vi "crc8.vi"(4 "Reflect Output? (F)":bool, 6 "Reflect Input? (F)":bool, 8 "Xor Out (0x00)":u8 format="%02x", 9 "Poly (0x07)":u8=7 format="%02x", 10 "Init (0x00)":u8 format="%02x", 11 "Data in":string) -> (3 "CRC-8":u8 format="%02x")   [LabVIEW 2021, in "hashlib.lvlib"]
doc: "Calculates a 8-bit Cyclic Redundancy Check (CRC-8) for various algorithms."
uses:
  hashlib.lvlib
panel:
  # "Data=\"123456789\"\n\nAlgorithm       CRC-8 Poly  Init  RefIn  RefOut XorOut\nCRC-8           0xF4  0x07  0x00  false  false  0x00\nCRC-8/CDMA2000  0xDA  0x9B  0xFF  false  false  0x00\nCRC-8/DARC      0x15  0x39  0x00  true   true   0x00\nCRC-8/DVB-S2    0xBC  0xD5  0x00  false  false  0x00\nCRC-8/EBU       0x97  0x1D  0xFF  true   true   0x00\nCRC-8/I-CODE    0x7E  0x1D  0xFD  false  false  0x00\nCRC-8/ITU       0xA1  0x07  0x00  false  false  0x55\nCRC-8/MAXIM     0xA1  0x31  0x00  true   true   0x00\nCRC-8/ROHC      0xD0  0x07  0xFF  true   true   0x00\nCRC-8/WCDMA     0x25  0x9B  0x00  true   true   0x00\n\nSource: https://crccalc.com/"
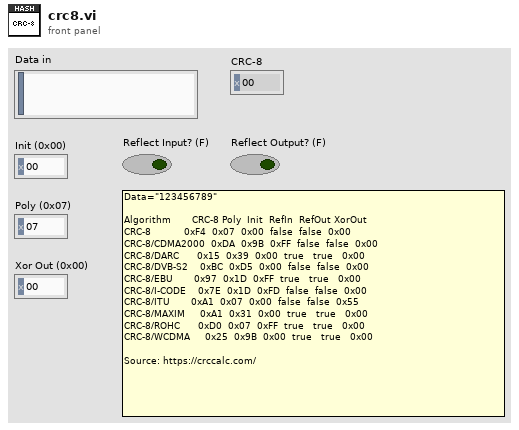
[diagram p1: front panel]
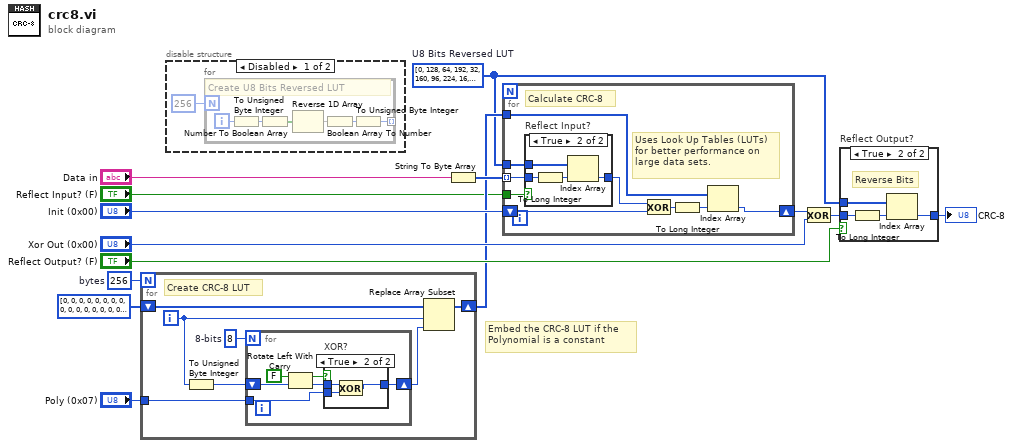
[diagram p0: block diagram]
diagram:
  w1 = u8[] [0, 128, 64, 192, 32, 160, 96, 224, 16, 144, 80, 208, 48, 176, 112, 240, 8, 136, 72, 200, 40, 168, 104, 232, 24, 152, 88, 216, 56, 184, 120, 248, 4, 132, 68, 196, 36, 164, 100, 228, 20, 148, 84, 212, 52, 180, 116, 244, 12, 140, 76, 204, 44, 172, 108, 236, 28, 156, 92, 220, 60, 188, 124, 252, 2, 130, 66, 194, 34, 162, 98, 226, 18, 146, 82, 210, 50, 178, 114, 242, 10, 138, 74, 202, 42, 170, 106, 234, 26, 154, 90, 218, 58, 186, 122, 250, 6, 134, 70, 198, 38, 166, 102, 230, 22, 150, 86, 214, 54, 182, 118, 246, 14, 142, 78, 206, 46, 174, 110, 238, 30, 158, 94, 222, 62, 190, 126, 254, 1, 129, 65, 193, 33, 161, 97, 225, 17, 145, 81, 209, 49, 177, 113, 241, 9, 137, 73, 201, 41, 169, 105, 233, 25, 153, 89, 217, 57, 185, 121, 249, 5, 133, 69, 197, 37, 165, 101, 229, 21, 149, 85, 213, 53, 181, 117, 245, 13, 141, 77, 205, 45, 173, 109, 237, 29, 157, 93, 221, 61, 189, 125, 253, 3, 131, 67, 195, 35, 163, 99, 227, 19, 147, 83, 211, 51, 179, 115, 243, 11, 139, 75, 203, 43, 171, 107, 235, 27, 155, 91, 219, 59, 187, 123, 251, 7, 135, 71, 199, 39, 167, 103, 231, 23, 151, 87, 215, 55, 183, 119, 247, 15, 143, 79, 207, 47, 175, 111, 239, 31, 159, 95, 223, 63, 191, 127, 255]  # U8 Bits Reversed LUT
  w8 = 256  # bytes
  # "Embed the CRC-8 LUT if the\nPolynomial is a constant"
  n1 = for {
    N: w8 -> [_]
    tunnel: "Poly (0x07)" -> [w20]
    shift-right: [w16] -> w3
    shift-left: u8[] [0, 0, 0, 0, 0, 0, 0, 0, 0, 0, 0, 0, 0, 0, 0, 0, 0, 0, 0, 0, 0, 0, 0, 0, 0, 0, 0, 0, 0, 0, 0, 0, 0, 0, 0, 0, 0, 0, 0, 0, 0, 0, 0, 0, 0, 0, 0, 0, 0, 0, 0, 0, 0, 0, 0, 0, 0, 0, 0, 0, 0, 0, 0, 0, 0, 0, 0, 0, 0, 0, 0, 0, 0, 0, 0, 0, 0, 0, 0, 0, 0, 0, 0, 0, 0, 0, 0, 0, 0, 0, 0, 0, 0, 0, 0, 0, 0, 0, 0, 0, 0, 0, 0, 0, 0, 0, 0, 0, 0, 0, 0, 0, 0, 0, 0, 0, 0, 0, 0, 0, 0, 0, 0, 0, 0, 0, 0, 0, 0, 0, 0, 0, 0, 0, 0, 0, 0, 0, 0, 0, 0, 0, 0, 0, 0, 0, 0, 0, 0, 0, 0, 0, 0, 0, 0, 0, 0, 0, 0, 0, 0, 0, 0, 0, 0, 0, 0, 0, 0, 0, 0, 0, 0, 0, 0, 0, 0, 0, 0, 0, 0, 0, 0, 0, 0, 0, 0, 0, 0, 0, 0, 0, 0, 0, 0, 0, 0, 0, 0, 0, 0, 0, 0, 0, 0, 0, 0, 0, 0, 0, 0, 0, 0, 0, 0, 0, 0, 0, 0, 0, 0, 0, 0, 0, 0, 0, 0, 0, 0, 0, 0, 0, 0, 0, 0, 0, 0, 0, 0, 0, 0, 0, 0, 0, 0, 0, 0, 0, 0, 0, 0, 0, 0, 0, 0, 0] -> [w19]
    i -> [w18]
    w21 = 8  # 8-bits
    # "Create CRC-8 LUT"
    n2 = To Unsigned Byte Integer(number=w18) -> (unsigned 8bit integer=w15:u8)
    n3 = for {
      N: w21 -> [_]
      shift-right: [w23] -> w17
      shift-left: w15 -> [w27]
      tunnel: w20 -> [w24]
      n4 = Rotate Left With Carry(2:w27, 3:FALSE ("carry")) -> (0:w25:u8, 1:w22:bool)
      n5 = case "XOR?" shown="True" w22 {
        tunnel: w25 -> [w28 w31]
        tunnel: w24 -> [_ w30]
        tunnel: [w28 w29] -> w23
        frame False {
        }
        frame True {
          n6 = Exclusive Or(1:w30, 2:w31) -> (0:w29:u8)
        }
      }
    }
    n7 = Replace Array Subset(array=w19, new element=w17, index=w18) -> (w16:u8[])
  }
  n8 = disable-structure shown="Disabled" {
    frame Disabled {
      n9 = for {
        N: 256 -> [_]
        tunnel: [w33] -> _ mode=indexing
        i -> [w38]
        # "Create U8 Bits Reversed LUT"
        n10 = To Unsigned Byte Integer(number=w38) -> (unsigned 8bit integer=w37:u8)
        n11 = Number To Boolean Array(number=w37) -> (Boolean array=w36:bool[])
        n12 = Reverse 1D Array(array=w36) -> (reversed array=w35:bool[])
        n13 = Boolean Array To Number(Boolean array=w35) -> (number=w34:u32)
        n14 = To Unsigned Byte Integer(number=w34) -> (unsigned 8bit integer=w33:u8)
      }
    }
    frame Enabled {
    }
  }
  n15 = String To Byte Array(string="Data in") -> (unsigned byte array=w7:u8[])
  n16 = for {
    shift-right: [w39] -> w6
    shift-left: "Init (0x00)" -> [w40]
    tunnel: w7 -> [w42] mode=indexing
    tunnel: w3 -> [w45]
    tunnel: "Reflect Input? (F)" -> [w41]
    tunnel: w1 -> [w44]
    # "Uses Look Up Tables (LUTs)\nfor better performance on\nlarge data sets."
    # "Calculate CRC-8"
    n17 = case "Reflect Input?" shown="True" w41 {
      tunnel: w42 -> [w48 w52]
      tunnel: w44 -> [_ w50]
      tunnel: [w48 w49] -> w43
      frame False {
      }
      frame True {
        n18 = To Long Integer(number=w52) -> (32bit integer=w51:i32)
        n19 = Index Array(array=w50, index=w51) -> (element=w49:u8)
      }
    }
    n20 = Exclusive Or(1:w40, 2:w43) -> (0:w47:u8)
    n21 = To Long Integer(number=w47) -> (32bit integer=w46:i32)
    n22 = Index Array(array=w45, index=w46) -> (element=w39:u8)
  }
  n23 = Exclusive Or(1:"Xor Out (0x00)", 2:w6) -> (0:w5:u8)
  n24 = case "Reflect Output?" shown="True" "Reflect Output? (F)" {
    tunnel: w5 -> [w53 w55]
    tunnel: [w53 w54] -> w13
    tunnel: w1 -> [_ w57]
    frame False {
    }
    frame True {
      # "Reverse Bits"
      n25 = To Long Integer(number=w55) -> (32bit integer=w56:i32)
      n26 = Index Array(array=w57, index=w56) -> (element=w54:u8)
    }
  }
  "CRC-8" <- w13
